vi "RSZVB Set SAW State.vi"(8 "error in (no error)":errorcluster {"code" format="%.0x"}, 9 "Apply (F: Off)":bool, 10 "Channel (1)":i32=1, 11 "VISA session":refnum<visa-resource-name>) -> (0 "error out":errorcluster {"code" format="%.0x"}, 3 "dup VISA session":refnum<visa-resource-name>)   [LabVIEW 2011]
doc: "This VI activates or deactivates the virtual matching network. When the network is activated, port 1 serves as an unbalanced port, the physical ports no. 2 and 3 of the analyzer are combined to a logical (balanced) port no. 2.\n\nRemote-control command(s):\nCALCulate<Ch>:FSIMulator:STATe ON | OFF"
panel:
  # "On\nOff"
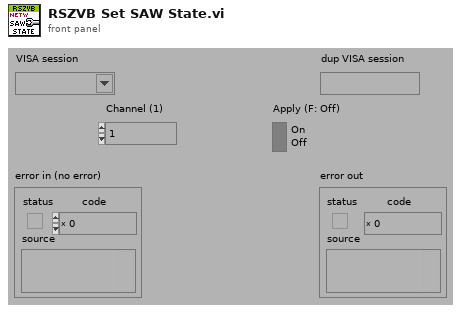
[diagram p1: front panel]
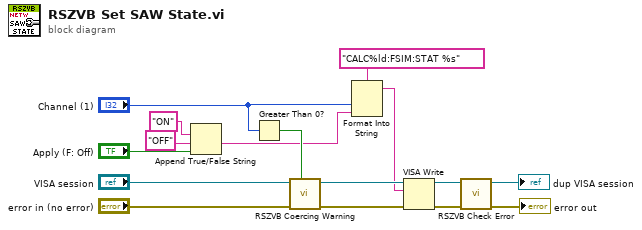
[diagram p0: block diagram]
diagram:
  n1 = Append True/False String(1:"Apply (F: Off)", 2:"OFF", 3:"ON") -> (0:w1:string)  [unwired: 1 in]
  n2 = Greater Than 0?(x="Channel (1)") -> (x > 0?=w8:bool)
  n3 = call "RSZVB Coercing Warning.vi"("In Range?"=w8, "error in (no error)"="error in (no error)", "VISA session"="VISA session") -> ("error out"=w14:errorcluster, "dup VISA session"=w15:refnum<visa-resource-name>)  [unwired: 7 in]
  n4 = Format Into String(format string="CALC%ld:FSIM:STAT %s", "Channel (1)", w1) -> (resulting string=w11:string)  [unwired: 2 in, 1 out]
  n5 = VISA Write(VISA resource name=w15, write buffer=w11, error in (no error)=w14) -> (VISA resource name out=w12:refnum<visa-resource-name>, error out=w13:errorcluster)  [unwired: 1 out]
  n6 = call "RSZVB Check Error.vi"("error in (no error)"=w13, "VISA session"=w12) -> ("error out"=→"error out":errorcluster, "dup VISA session"=→"dup VISA session":refnum<visa-resource-name>)  [unwired: 8 in]
